vi "MSR Main.vi"() -> ()   [LabVIEW 2019]
uses:
  <vilib>/Platform/TimedLoop/XDataNode/timing_clust.ctl
  <vilib>/Platform/TimedLoop/XDataNode/nitl_modes.ctl
  <vilib>/Platform/TimedLoop/XDataNode/wakeup.ctl
  <vilib>/platform/TimedLoop/XDataNode/XDataNode.xnode
  <vilib>/Platform/TimedLoop/XDataNode/XDNodeRunTimeDep.lvlib
panel:
  in  "Tab Control":enum32{"Plots", "Debug"}(tab)
  out "Flow Plot":cluster{dbl[], dbl[]}(graph)
  out "Temperature Plot":cluster{dbl[], dbl[]}[](graph)
  in  "?":u16(ring)=3 items=["Primary Temperatures", "Secondary Temperatures", "Air Temperatures", "Pri and Sec Temperatures"]
  in  "?":u16(ring) items=["Primary Flow", "Secondary Flow", "Air Flow"]
  out "PriLoops":i32=318
  out "MainLoops":i32=318
  out "SecLoops":i32=318
  out "Time Interval (s)":dbl=0.002
  out "AirLoops":i32=318
  out "Running":bool=TRUE
  out "MHX Heat Transfer (W)":dbl=29227.364495201997 format="%#.0f"
  in  "Period (ms)":i64=2
  out "NDHX Heat Transfer (W)":dbl
  in  "Speed":u16(ring) items=["1x", "10x", "100x", "250x"]
  out "Time Elapsed (s)":dbl=0.6360000000000005
  out "Primary Flow (kg/s)":dbl=0.15588909681163526 format="%.2f"
  out "Primary Cold Temperature (C)":dbl=509.9990851167456 format="%#.1f"
  out "Primary Hot Temperature (C)":dbl=530.011541963479 format="%#.1f"
  out "Primary Ave Temperature (C)":dbl=520.0052977887772 format="%#.1f"
  out "Secondary Flow (kg/s)":dbl=0.18722572734626322 format="%.2f"
  out "Secondary Hot Temperature (C)":dbl=501.012014998414 format="%#.1f"
  out "Secondary Cold Temperature (C)":dbl=490.0008668458488 format="%#.1f"
  out "Secondary Ave Temperature (C)":dbl=495.5064099599597 format="%#.1f"
  out "Air Flow (kg/s)":dbl=0.0013110826649570554 format="%.2f"
  in  "Louver Position (% Open)":dbl=35.0 min=0.0 max=100.0
  in  "Reactor Power (W)":dbl=200000.0 min=0.0 max=250000.0
  out "Air Ave Temperature (C)":dbl=20.007970254732186 format="%#.1f"
  out "Air Outlet Temperature (C)":dbl=20.015996677171586 format="%#.1f"
  in  "Stop":bool
  in  "Air Inlet Temperature (C)":dbl=20.0 min=-89.0 max=57.0
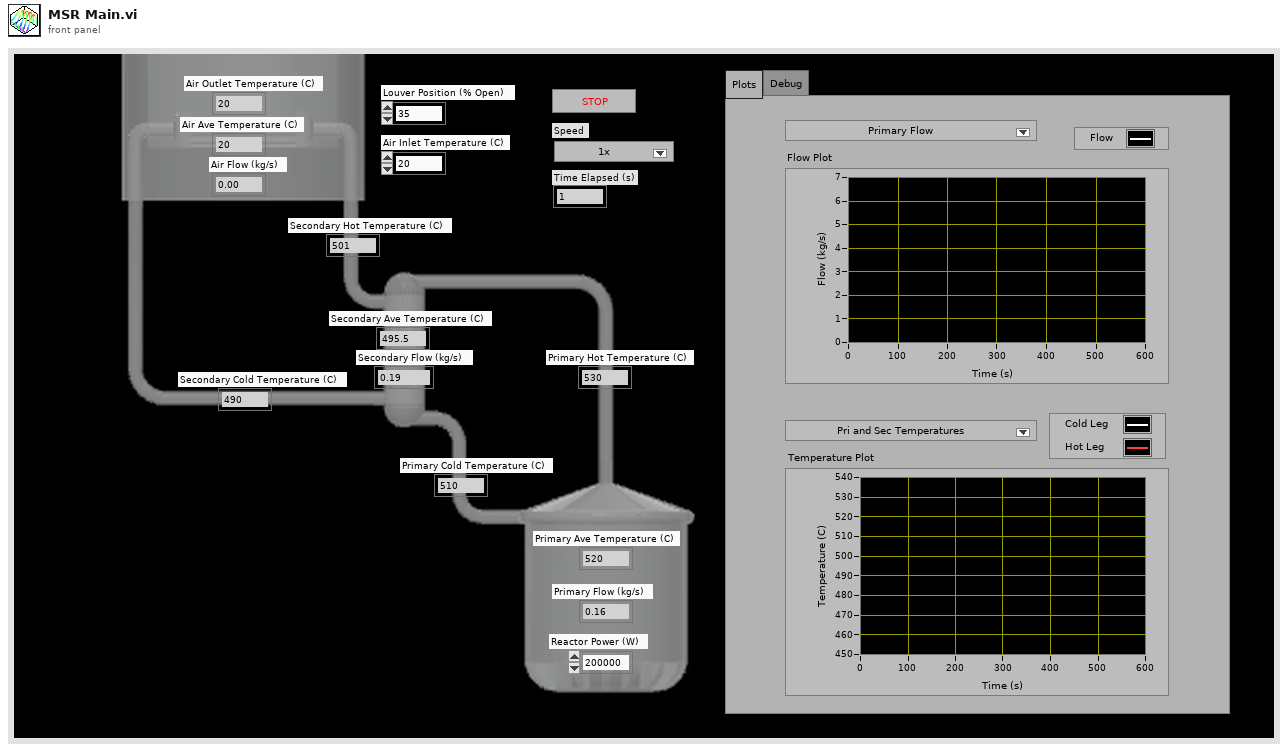
[diagram p1: front panel]
types:
  T1 = cluster{"Air Queue":refnum<queue>, "Air Err":errorcluster, "Pri Queue":refnum<queue>, "Sec Queue":refnum<queue>, "Pri Err":errorcluster, "Sec Err":errorcluster}
  T2 = cluster{"Air Outlet Temperature (K)":dbl, "Air Flow (kg/s)":dbl, "NDHX Wall Temperature (K)":dbl, "Air Visc (Pa-s)":dbl, "Pri Flow (kg/s)":dbl, "Pri Hot Temp (K)":dbl, "Pri Cold Temp (K)":dbl, "Sec Flow (kg/s)":dbl, "Sec Hot Temp (K)":dbl, "Sec Cold Temp (K)":dbl, "MHX Wall Temp (K)":dbl, "FLiNaK Visc (Pa-s)":dbl}
  T3 = cluster{"Pri Flow (kg/s)":dbl, "Pri Hot Temp (K)":dbl, "Pri Cold Temp (K)":dbl}
  T4 = cluster{"Sec Flow (kg/s)":dbl, "Sec Hot Temp (K)":dbl, "Sec Cold Temp (K)":dbl, "MHX Wall Temp (K)":dbl, "FLiNaK Visc (Pa-s)":dbl}
  T5 = typedef "XDNodeRunTimeDep.lvlib/timing_clust.ctl" = cluster{"Expected End [f-1]":u64, "Actual End [f-1]":u64, "Finished Late? [f-1]":bool, "Expected End [i-1]":u64, "Actual End [i-1]":u64, "Finished Late? [i-1]":bool, "Expected Start [i]":u64, "Actual Start [i]":u64, "Expected Start [f]":u64, "Actual Start [f]":u64, "Source Name":string, "Structure Name":string, "Period":i64, "Deadline":i64, "Offset":i64, "Start":i64, "Priority":i32, "Timeout":i32, "Mode":T6, "Wakeup Reason":T7, "Error":errorcluster, "Source Type":string, "Secondary Source Type":string, "Global End Time":u64, "Global Start Time":u64, "Frame Duration":u64, "Iteration Duration":u64, "Assigned CPU":i32, "I/O Scan Engine Mode":u32}
  T6 = typedef "XDNodeRunTimeDep.lvlib/nitl_modes.ctl" = enum32{"No Change", "Process missed periods, maintain original phase", "Discard missed periods, maintain original phase", "Process missed periods, ignore original phase", "Discard missed periods, ignore original phase"}
  T7 = typedef "XDNodeRunTimeDep.lvlib/wakeup.ctl" = enum32{"Normal", "Aborted", "Asynchronous wakeup", "Timing source error", "Timed loop error", "Timeout"}
  T8 = cluster{"Air Outlet Temperature (K)":dbl, "Air Flow (kg/s)":dbl, "NDHX Wall Temperature (K)":dbl, "Air Visc (Pa-s)":dbl}
  T9 = cluster{"Time (s)":dbl, "Air Flow (kg/s)":dbl, "Air Outlet Temp (C)":dbl, "Air Inlet Temp (C)":dbl, "Sec Hot Temp (C)":dbl, "Sec Cold Temp (C)":dbl, "Sec Flow (kg/s)":dbl, "Pri Flow (kg/s)":dbl, "Pri Hot Temp (C)":dbl, "Pri Cold Temp (C)":dbl}
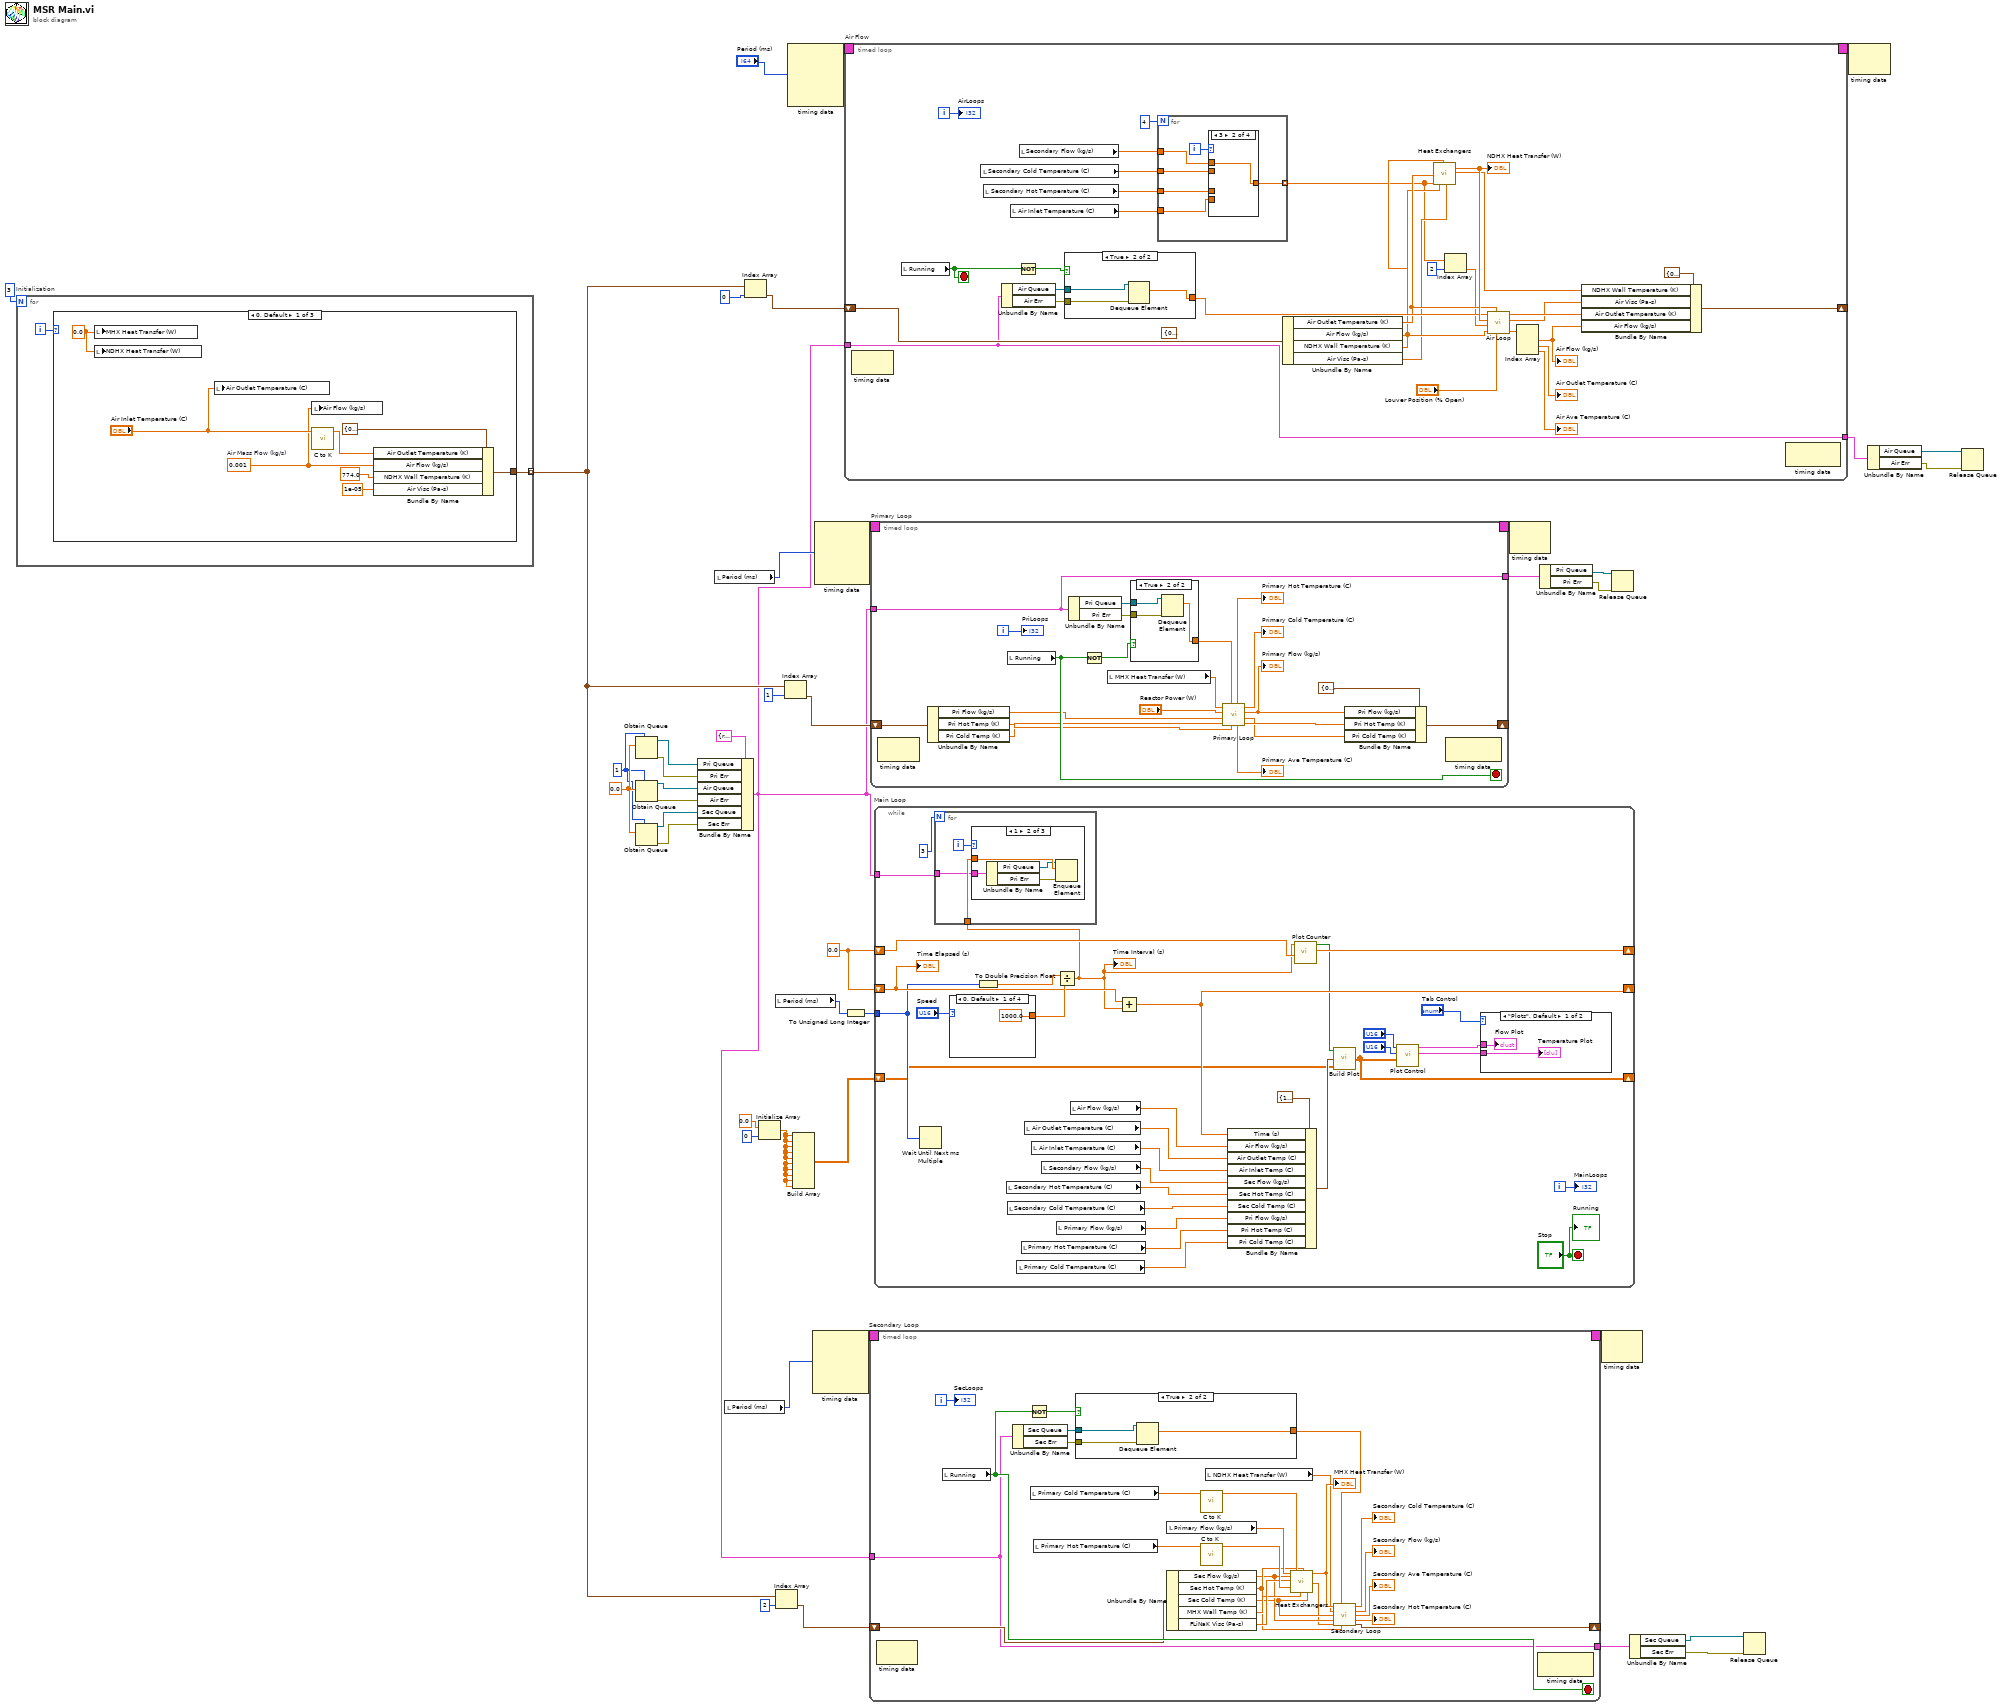
[diagram p0: block diagram]
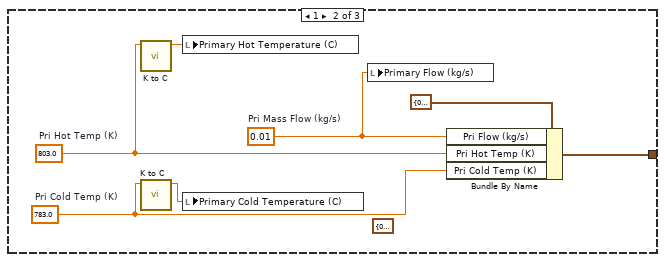
[diagram p2: hidden frame]
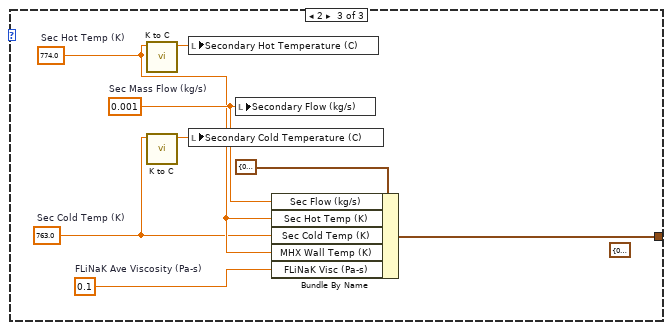
[diagram p3: hidden frame]
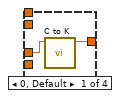
[diagram p4: hidden frame]
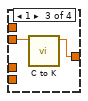
[diagram p5: hidden frame]
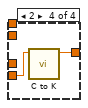
[diagram p6: hidden frame]
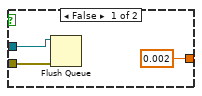
[diagram p7: hidden frame]
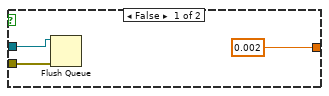
[diagram p8: hidden frame]
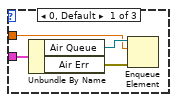
[diagram p9: hidden frame]
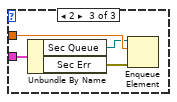
[diagram p10: hidden frame]
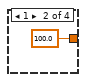
[diagram p12: hidden frame]
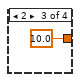
[diagram p13: hidden frame]
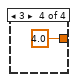
[diagram p14: hidden frame]
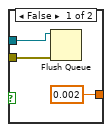
[diagram p15: hidden frame]
diagram:
  w10 = 1 ("max queue size (-1, unlimited)")
  w30 = 0.0
  w35 = 0.0
  n1 = for "Initialization" {
    N: 3 -> [_]
    tunnel: [w45] -> w22 mode=indexing
    i -> [w44]
    n2 = case shown="0, Default" w44 {
      tunnel: [w47 w55 w62] -> w45
      frame 0, Default {
        w46 = 0.0 ("NDHX Heat Transfer (W)")
        w50 = 0.001  # Air Mass Flow (kg/s)
        n3 = local write "MHX Heat Transfer (W)"(w46) -> ()
        n4 = local write "NDHX Heat Transfer (W)"(w46) -> ()
        n5 = local write "Air Outlet Temperature (C)"("Air Inlet Temperature (C)") -> ()
        n6 = local write "Air Flow (kg/s)"(w50) -> ()
        n7 = call "C to K.vi"("Temperature (C)"="Air Inlet Temperature (C)") -> ("Temperature (K)"=w53:dbl)  [unwired: 10 in]
        n8 = Bundle By Name(cluster=T2 {"Air Outlet Temperature (K)"=0.0, "Air Flow (kg/s)"=0.0, "NDHX Wall Temperature (K)"=0.0, "Air Visc (Pa-s)"=0.0, "Pri Flow (kg/s)"=0.0, "Pri Hot Temp (K)"=0.0, "Pri Cold Temp (K)"=0.0, "Sec Flow (kg/s)"=0.0, "Sec Hot Temp (K)"=0.0, "Sec Cold Temp (K)"=0.0, "MHX Wall Temp (K)"=0.0, "FLiNaK Visc (Pa-s)"=0.0} ("input cluster"), "Air Outlet Temperature (K)"=w53, "Air Flow (kg/s)"=w50, "NDHX Wall Temperature (K)"=774.0, "Air Visc (Pa-s)"=1e-05 ("Air Average Viscosity (Pa-s)")) -> (w47:T2)
      }
      frame 1 {
        (unwired) T3 {"Pri Flow (kg/s)"=0.0, "Pri Hot Temp (K)"=0.0, "Pri Cold Temp (K)"=0.0} ("input cluster")
        w58 = 0.01  # Pri Mass Flow (kg/s)
        w56 = 783.0  # Pri Cold Temp (K)
        w57 = 803.0  # Pri Hot Temp (K)
        n9 = call "K to C.vi"("Temperature (K)"=w57) -> ("Temperature (C)"=w60:dbl)  [unwired: 10 in]
        n10 = call "K to C.vi"("Temperature (K)"=w56) -> ("Temperature (C)"=w59:dbl)  [unwired: 10 in]
        n11 = local write "Primary Hot Temperature (C)"(w60) -> ()
        n12 = local write "Primary Cold Temperature (C)"(w59) -> ()
        n13 = local write "Primary Flow (kg/s)"(w58) -> ()
        n14 = Bundle By Name(cluster=T2 {"Air Outlet Temperature (K)"=0.0, "Air Flow (kg/s)"=0.0, "NDHX Wall Temperature (K)"=0.0, "Air Visc (Pa-s)"=0.0, "Pri Flow (kg/s)"=0.0, "Pri Hot Temp (K)"=0.0, "Pri Cold Temp (K)"=0.0, "Sec Flow (kg/s)"=0.0, "Sec Hot Temp (K)"=0.0, "Sec Cold Temp (K)"=0.0, "MHX Wall Temp (K)"=0.0, "FLiNaK Visc (Pa-s)"=0.0} ("input cluster"), "Pri Flow (kg/s)"=w58, "Pri Hot Temp (K)"=w57, "Pri Cold Temp (K)"=w56) -> (w55:T2)
      }
      frame 2 {
        (unwired) T4 {"Sec Flow (kg/s)"=0.0, "Sec Hot Temp (K)"=0.0, "Sec Cold Temp (K)"=0.0, "MHX Wall Temp (K)"=0.0, "FLiNaK Visc (Pa-s)"=0.0} ("input cluster")
        w63 = 0.1  # FLiNaK Ave Viscosity (Pa-s)
        w66 = 0.001  # Sec Mass Flow (kg/s)
        w64 = 763.0  # Sec Cold Temp (K)
        w65 = 774.0  # Sec Hot Temp (K)
        n15 = call "K to C.vi"("Temperature (K)"=w65) -> ("Temperature (C)"=w68:dbl)  [unwired: 10 in]
        n16 = call "K to C.vi"("Temperature (K)"=w64) -> ("Temperature (C)"=w67:dbl)  [unwired: 10 in]
        n17 = local write "Secondary Hot Temperature (C)"(w68) -> ()
        n18 = local write "Secondary Cold Temperature (C)"(w67) -> ()
        n19 = local write "Secondary Flow (kg/s)"(w66) -> ()
        n20 = Bundle By Name(cluster=T2 {"Air Outlet Temperature (K)"=0.0, "Air Flow (kg/s)"=0.0, "NDHX Wall Temperature (K)"=0.0, "Air Visc (Pa-s)"=0.0, "Pri Flow (kg/s)"=0.0, "Pri Hot Temp (K)"=0.0, "Pri Cold Temp (K)"=0.0, "Sec Flow (kg/s)"=0.0, "Sec Hot Temp (K)"=0.0, "Sec Cold Temp (K)"=0.0, "MHX Wall Temp (K)"=0.0, "FLiNaK Visc (Pa-s)"=0.0} ("input cluster"), "Sec Flow (kg/s)"=w66, "Sec Hot Temp (K)"=w65, "Sec Cold Temp (K)"=w64, "MHX Wall Temp (K)"=w65, "FLiNaK Visc (Pa-s)"=w63) -> (w62:T2)
      }
    }
  }
  n21 = Obtain Queue(max queue size (-1, unlimited)=w10, element data type=w35) -> (queue out=w18:refnum<queue>, error out=w17:errorcluster)  [unwired: 3 in, 1 out]
  n22 = Obtain Queue(max queue size (-1, unlimited)=w10, element data type=w35) -> (queue out=w16:refnum<queue>, error out=w15:errorcluster)  [unwired: 3 in, 1 out]
  n23 = Obtain Queue(max queue size (-1, unlimited)=w10, element data type=w35) -> (queue out=w14:refnum<queue>, error out=w13:errorcluster)  [unwired: 3 in, 1 out]
  n24 = Bundle By Name(cluster=T1 {"Air Queue"=refnum, "Air Err"={"status"=FALSE, "code"=0, "source"=""}, "Pri Queue"=refnum, "Sec Queue"=refnum, "Pri Err"={"status"=FALSE, "code"=0, "source"=""}, "Sec Err"={"status"=FALSE, "code"=0, "source"=""}} ("input cluster"), "Pri Queue"=w18, "Pri Err"=w17, "Air Queue"=w16, "Air Err"=w15, "Sec Queue"=w14, "Sec Err"=w13) -> (w11:T1)
  n25 = local read "Period (ms)"() -> (w21:i64)
  n26 = local read "Period (ms)"() -> (w19:i64)
  n27 = Index Array(array=w22, index=0) -> (element=w26:T2)
  n28 = Initialize Array(0.0 ("element"), 0 ("dimension size")) -> (w32:dbl[])
  n29 = local read "Period (ms)"() -> (w20:i64)
  n30 = Index Array(array=w22, index=2) -> (element=w23:T2)
  n31 = Index Array(array=w22, index=1) -> (element=w27:T2)
  n32 = node-c288("Period (ms)") -> (w38:T5)  [unwired: 3 in]
  n33 = Build Array(w32, w32, w32, w32, w32, w32, w32, w32, w32, w32) -> (w31:dbl[][])
  n34 = node-c288(w19) -> (w41:T5)  [unwired: 3 in]
  n35 = node-c288(w21) -> (w43:T5)  [unwired: 3 in]
  n36 = timed-loop "Air Flow" {
    timing: w38 -> [_]
    timing-out: [_] -> w37
    shift-right: [w80] -> _
    shift-left: w26 -> [w93]
    tunnel: w11 -> [w77]
    tunnel: [w77] -> w7
    i -> [w99]
    stop <- w96 stop-if-true
    (unwired) T8 {"Air Outlet Temperature (K)"=0.0, "Air Flow (kg/s)"=0.0, "NDHX Wall Temperature (K)"=0.0, "Air Visc (Pa-s)"=0.0} ("input cluster")
    n37 = node-c288() -> ()  [unwired: 1 in, 1 out]
    n38 = local read "Running"() -> (w96:bool)
    n39 = local read "Secondary Cold Temperature (C)"() -> (w87:dbl)
    n40 = local read "Secondary Hot Temperature (C)"() -> (w88:dbl)
    n41 = Unbundle By Name(w77) -> ("Air Queue"=w79:refnum<queue>, "Air Err"=w78:errorcluster)
    n42 = local read "Air Inlet Temperature (C)"() -> (w86:dbl)
    n43 = Not(x=w96) -> (.not. x?=w98:bool)
    n44 = local read "Secondary Flow (kg/s)"() -> (w69:dbl)
    n45 = case shown="True" w98 {
      tunnel: w79 -> [w115 w117]
      tunnel: w78 -> [w114 w116]
      tunnel: [0.002 w118] -> w94
      frame False {
        n46 = Flush Queue(queue=w115, error in (no error)=w114) -> ()  [unwired: 3 out]
      }
      frame True {
        n47 = Dequeue Element(queue=w117, error in (no error)=w116) -> (element=w118:dbl)  [unwired: 1 in, 3 out]
      }
    }
    n48 = for {
      N: 4 -> [_]
      tunnel: w88 -> [w104]
      tunnel: w87 -> [w102]
      tunnel: w86 -> [w101]
      tunnel: [w103] -> w82 mode=indexing
      tunnel: w69 -> [w100]
      i -> [w105]
      n49 = case shown="3" w105 {
        tunnel: w104 -> [w107 _ _ _]
        tunnel: [w106 w108 w109 w111] -> w103
        tunnel: w102 -> [_ _ w110 _]
        tunnel: w101 -> [_ _ _ w112]
        tunnel: w100 -> [_ w108 _ _]
        frame 0, Default {
          n50 = call "C to K.vi"("Temperature (C)"=w107) -> ("Temperature (K)"=w106:dbl)  [unwired: 10 in]
        }
        frame 3 {
        }
        frame 1 {
          n51 = call "C to K.vi"("Temperature (C)"=w110) -> ("Temperature (K)"=w109:dbl)  [unwired: 10 in]
        }
        frame 2 {
          n52 = call "C to K.vi"("Temperature (C)"=w112) -> ("Temperature (K)"=w111:dbl)  [unwired: 10 in]
        }
      }
    }
    n53 = Unbundle By Name(w93) -> ("Air Outlet Temperature (K)"=w92:dbl, "Air Flow (kg/s)"=w91:dbl, "NDHX Wall Temperature (K)"=w90:dbl, "Air Visc (Pa-s)"=w89:dbl)
    n54 = call "Heat Exchangers.vi"("Air Hot Temperature (K), N"=w92, "Local Array In, N"=w82, "NDHX Tube Wall Temp (K), N"=w90, "Air Flow (kg/s), N"=w91, "Air Average Viscosity (Pa-s), N"=w89) -> ("NDHX Heating Transfer (W)"=w95:dbl, "NDHX Tube Wall Temperature (K)"=w76:dbl)  [unwired: 11 in, 2 out]
    "NDHX Heat Transfer (W)" <- w95
    n55 = Index Array(array=w82, index=2) -> (element=w83:dbl)
    n56 = call "Air Loop.vi"("Louver Position (% Open)"="Louver Position (% Open)", "Air Hot Temperature (K)"=w92, "Air Mass Flow (kg/s) in"=w91, "Air Inlet Temperature (K)"=w83, "NDHX Heat Transfer (W)"=w95, "Time Interval (s)"=w94) -> ("Indications"=w75:dbl[], "Air Average Viscosity (Pa-s)"=w71:dbl, "Air Outlet Temperature (K)"=w72:dbl)  [unwired: 2 in, 1 out]
    n57 = Index Array(array=w75) -> (element #1=w70:dbl, element #2=→"Air Outlet Temperature (C)":dbl, element #3=→"Air Ave Temperature (C)":dbl)  [unwired: 3 in]
    "Air Flow (kg/s)" <- w70
    n58 = Bundle By Name(cluster=T2 {"Air Outlet Temperature (K)"=0.0, "Air Flow (kg/s)"=0.0, "NDHX Wall Temperature (K)"=0.0, "Air Visc (Pa-s)"=0.0, "Pri Flow (kg/s)"=0.0, "Pri Hot Temp (K)"=0.0, "Pri Cold Temp (K)"=0.0, "Sec Flow (kg/s)"=0.0, "Sec Hot Temp (K)"=0.0, "Sec Cold Temp (K)"=0.0, "MHX Wall Temp (K)"=0.0, "FLiNaK Visc (Pa-s)"=0.0} ("input cluster"), "NDHX Wall Temperature (K)"=w76, "Air Visc (Pa-s)"=w71, "Air Outlet Temperature (K)"=w72, "Air Flow (kg/s)"=w70) -> (w80:T2)
    n59 = node-c288() -> ()  [unwired: 1 in, 1 out]
    "AirLoops" <- w99
  }
  n60 = To Unsigned Long Integer(number=w20) -> (unsigned 32bit integer=w39:u32)
  n61 = timed-loop "Secondary Loop" {
    timing: w41 -> [_]
    timing-out: [_] -> w40
    shift-right: [w125] -> _
    shift-left: w23 -> [w134]
    tunnel: w11 -> [w122]
    tunnel: [w122] -> w3
    i -> [w146]
    stop <- w144 stop-if-true
    n62 = node-c288() -> ()  [unwired: 1 in, 1 out]
    n63 = local read "Running"() -> (w144:bool)
    n64 = Unbundle By Name(w122) -> ("Sec Queue"=w124:refnum<queue>, "Sec Err"=w123:errorcluster)
    n65 = Not(x=w144) -> (.not. x?=w143:bool)
    n66 = local read "Primary Cold Temperature (C)"() -> (w140:dbl)
    n67 = local read "Primary Hot Temperature (C)"() -> (w141:dbl)
    n68 = case shown="True" w143 {
      tunnel: w124 -> [w149 w152]
      tunnel: w123 -> [w148 w151]
      tunnel: [0.002 w150] -> w136
      frame False {
        n69 = Flush Queue(queue=w149, error in (no error)=w148) -> ()  [unwired: 3 out]
      }
      frame True {
        n70 = Dequeue Element(queue=w152, error in (no error)=w151) -> (element=w150:dbl)  [unwired: 1 in, 3 out]
      }
    }
    n71 = local read "Primary Flow (kg/s)"() -> (w142:dbl)
    n72 = Unbundle By Name(w134) -> ("Sec Flow (kg/s)"=w130:dbl, "Sec Hot Temp (K)"=w131:dbl, "Sec Cold Temp (K)"=w129:dbl, "MHX Wall Temp (K)"=w132:dbl, "FLiNaK Visc (Pa-s)"=w133:dbl)
    n73 = call "C to K.vi"("Temperature (C)"=w140) -> ("Temperature (K)"=w139:dbl)  [unwired: 10 in]
    n74 = call "C to K.vi"("Temperature (C)"=w141) -> ("Temperature (K)"=w138:dbl)  [unwired: 10 in]
    n75 = local read "NDHX Heat Transfer (W)"() -> (w121:dbl)
    n76 = call "Heat Exchangers.vi"("Primary Flow (kg/s), M"=w142, "Secondary Flow (kg/s)"=w130, "FLiNaK Ave Viscosity (Pa-s), M"=w133, "Pri Hot Temperature (K), M"=w138, "Pri Cold Temperature (K), M"=w139, "MHX Tube Wall Temp (K), M"=w132, "Sec Hot Temperature (K)"=w131, "Sec Cold Temperature (K)"=w129) -> ("MHX Heat Transfer (W)"=w137:dbl, "MHX Tube Wall Temperature (K)"=w128:dbl)  [unwired: 8 in, 2 out]
    "MHX Heat Transfer (W)" <- w137
    n77 = call "Secondary Loop.vi"("MHX Heat Transfer (W)"=w137, "Time Interval (s)"=w136, "NDHX Heat Transfer (W)"=w121, "Sec Cold Temp (K)"=w129, "Sec Mass Flow (kg/s) in"=w130, "MHX Wall Temp (K)"=w128, "Sec Hot Temp (K) in"=w131) -> ("Sec Cold Temperature (C)"=→"Secondary Cold Temperature (C)":dbl, "Sec Mass Flow (kg/s) out"=→"Secondary Flow (kg/s)":dbl, "Secondary Average Temperature (C)"=→"Secondary Ave Temperature (C)":dbl, "Sec Hot Temperature (C)"=→"Secondary Hot Temperature (C)":dbl, "output cluster"=w125:T2)  [unwired: 4 in]
    n78 = node-c288() -> ()  [unwired: 1 in, 1 out]
    "SecLoops" <- w146
  }
  n79 = timed-loop "Primary Loop" {
    timing: w43 -> [_]
    timing-out: [_] -> w42
    shift-right: [w158] -> _
    shift-left: w27 -> [w163]
    tunnel: w11 -> [w155]
    tunnel: [w155] -> w6
    i -> [w175]
    stop <- w170 stop-if-true
    n80 = node-c288() -> ()  [unwired: 1 in, 1 out]
    n81 = Unbundle By Name(w163) -> ("Pri Flow (kg/s)"=w162:dbl, "Pri Hot Temp (K)"=w161:dbl, "Pri Cold Temp (K)"=w160:dbl)
    n82 = local read "Running"() -> (w170:bool)
    n83 = Unbundle By Name(w155) -> ("Pri Queue"=w157:refnum<queue>, "Pri Err"=w156:errorcluster)
    n84 = Not(x=w170) -> (.not. x?=w169:bool)
    n85 = local read "MHX Heat Transfer (W)"() -> (w168:dbl)
    n86 = case shown="True" w169 {
      tunnel: w157 -> [w178 w180]
      tunnel: w156 -> [w177 w179]
      tunnel: [0.002 w181] -> w167
      frame False {
        n87 = Flush Queue(queue=w178, error in (no error)=w177) -> ()  [unwired: 3 out]
      }
      frame True {
        n88 = Dequeue Element(queue=w180, error in (no error)=w179) -> (element=w181:dbl)  [unwired: 1 in, 3 out]
      }
    }
    n89 = call "Primary Loop.vi"("Pri Hot Temp (K)"=w161, "Time Interval (s)"=w167, "Pri Cold Temp (K)"=w160, "Pri Mass Flow (kg/s) in"=w162, "Reactor Power (W)"="Reactor Power (W)", "MHX Heat Transfer (W)"=w168) -> ("Pri Hot Temperature (K)"=w165:dbl, "Pri Cold Temperature (K)"=w164:dbl, "Pri Mass Flow (kg/s) out"=w166:dbl, "Temperature (C) 2"=→"Primary Cold Temperature (C)":dbl, "Primary Average Temperature (C)"=→"Primary Ave Temperature (C)":dbl, "Temperature (C)"=→"Primary Hot Temperature (C)":dbl)
    "Primary Flow (kg/s)" <- w166
    n90 = Bundle By Name(cluster=T2 {"Air Outlet Temperature (K)"=0.0, "Air Flow (kg/s)"=0.0, "NDHX Wall Temperature (K)"=0.0, "Air Visc (Pa-s)"=0.0, "Pri Flow (kg/s)"=0.0, "Pri Hot Temp (K)"=0.0, "Pri Cold Temp (K)"=0.0, "Sec Flow (kg/s)"=0.0, "Sec Hot Temp (K)"=0.0, "Sec Cold Temp (K)"=0.0, "MHX Wall Temp (K)"=0.0, "FLiNaK Visc (Pa-s)"=0.0} ("input cluster"), "Pri Flow (kg/s)"=w166, "Pri Hot Temp (K)"=w165, "Pri Cold Temp (K)"=w164) -> (w158:T2)
    n91 = node-c288() -> ()  [unwired: 1 in, 1 out]
    "PriLoops" <- w175
  }
  n92 = while "Main Loop" {
    shift-right: [w200] -> _
    shift-left: w30 -> [w212]
    shift-right: [w208] -> _
    shift-left: w30 -> [w203]
    tunnel: w39 -> [w207]
    shift-right: [w186] -> _
    shift-left: w31 -> [w187]
    tunnel: w11 -> [w185]
    i -> [w209]
    stop <- "Stop" stop-if-true
    n93 = Wait Until Next ms Multiple(millisecond multiple=w207) -> ()  [unwired: 1 out]
    n94 = case shown="0, Default" "Speed" {
      tunnel: [1000.0 100.0 ("y") 10.0 ("y") 4.0 ("y")] -> w213
      frame 0, Default {
      }
      frame 1 {
      }
      frame 2 {
      }
      frame 3 {
      }
    }
    n95 = To Double Precision Float(number=w207) -> (double precision float=w215:dbl)
    n96 = local read "Secondary Hot Temperature (C)"() -> (w195:dbl)
    n97 = local read "Secondary Cold Temperature (C)"() -> (w194:dbl)
    n98 = local read "Primary Cold Temperature (C)"() -> (w191:dbl)
    n99 = local read "Primary Hot Temperature (C)"() -> (w192:dbl)
    n100 = local read "Air Outlet Temperature (C)"() -> (w198:dbl)
    n101 = local read "Air Inlet Temperature (C)"() -> (w197:dbl)
    n102 = local read "Secondary Flow (kg/s)"() -> (w196:dbl)
    n103 = Divide(x=w215, y=w213) -> (x/y=w202:dbl)
    "Time Interval (s)" <- w202
    n104 = for {
      N: 3 -> [_]
      tunnel: w202 -> [w218]
      tunnel: w185 -> [w217]
      i -> [w216]
      n105 = case shown="1" w216 {
        tunnel: w218 -> [w219 w226 w230]
        tunnel: w217 -> [w220 w225 w229]
        frame 0, Default {
          n106 = Unbundle By Name(w220) -> ("Air Queue"=w222:refnum<queue>, "Air Err"=w221:errorcluster)
          n107 = Enqueue Element(queue=w222, element=w219, error in (no error)=w221) -> ()  [unwired: 1 in, 3 out]
        }
        frame 1 {
          n108 = Unbundle By Name(w225) -> ("Pri Queue"=w224:refnum<queue>, "Pri Err"=w223:errorcluster)
          n109 = Enqueue Element(queue=w224, element=w226, error in (no error)=w223) -> ()  [unwired: 1 in, 3 out]
        }
        frame 2 {
          n110 = Unbundle By Name(w229) -> ("Sec Queue"=w228:refnum<queue>, "Sec Err"=w227:errorcluster)
          n111 = Enqueue Element(queue=w228, element=w230, error in (no error)=w227) -> ()  [unwired: 1 in, 3 out]
        }
      }
    }
    n112 = local read "Primary Flow (kg/s)"() -> (w193:dbl)
    n113 = local read "Air Flow (kg/s)"() -> (w199:dbl)
    n114 = Add(x=w212, y=w202) -> (x+y=w200:dbl)
    n115 = Bundle By Name(cluster=T9 {"Time (s)"=1000.0, "Air Flow (kg/s)"=1000.0, "Air Outlet Temp (C)"=1000.0, "Air Inlet Temp (C)"=1000.0, "Sec Hot Temp (C)"=1000.0, "Sec Cold Temp (C)"=1000.0, "Sec Flow (kg/s)"=1000.0, "Pri Flow (kg/s)"=1000.0, "Pri Hot Temp (C)"=1000.0, "Pri Cold Temp (C)"=1000.0} ("input cluster"), "Time (s)"=w200, "Air Flow (kg/s)"=w199, "Air Outlet Temp (C)"=w198, "Air Inlet Temp (C)"=w197, "Sec Flow (kg/s)"=w196, "Sec Hot Temp (C)"=w195, "Sec Cold Temp (C)"=w194, "Pri Flow (kg/s)"=w193, "Pri Hot Temp (C)"=w192, "Pri Cold Temp (C)"=w191) -> (w188:T9)
    n116 = call "Plot Counter.vi"("y in"=w203, "Numeric"=w202) -> ("y out"=w208:dbl, "Boolean out"=w189:bool)  [unwired: 8 in]
    n117 = call "Build Plot.vi"("Array in"=w187, "Data cluster"=w188, "Boolean in"=w189) -> ("Array out"=w186:dbl[][])
    n118 = call "Plot Control.vi"("Data"=w186, "Temperature Selection"="?", "Flow Selection"="?") -> ("Temperature Plot"=w204:cluster{"Array out":dbl[], "Array out":dbl[]}[], "Flow Plot"=w205:cluster{"Array out":dbl[], "Array out":dbl[]})  [unwired: 7 in]
    n119 = case shown="\"Plots\", Default" "Tab Control" {
      tunnel: w205 -> [w232 _]
      tunnel: w204 -> [w231 _]
      frame "Plots", Default {
        "Flow Plot" <- w232
        "Temperature Plot" <- w231
      }
      frame "Debug" {
      }
    }
    "Time Elapsed (s)" <- w212
    "MainLoops" <- w209
    "Running" <- "Stop"
  }
  n120 = node-c288(w42) -> ()  [unwired: 1 out]
  n121 = Unbundle By Name(w6) -> ("Pri Queue"=w5:refnum<queue>, "Pri Err"=w4:errorcluster)
  n122 = node-c288(w40) -> ()  [unwired: 1 out]
  n123 = Release Queue(queue=w5, error in (no error)=w4) -> ()  [unwired: 1 in, 3 out]
  n124 = Unbundle By Name(w3) -> ("Sec Queue"=w2:refnum<queue>, "Sec Err"=w1:errorcluster)
  n125 = Release Queue(queue=w2, error in (no error)=w1) -> ()  [unwired: 1 in, 3 out]
  n126 = node-c288(w37) -> ()  [unwired: 1 out]
  n127 = Unbundle By Name(w7) -> ("Air Queue"=w9:refnum<queue>, "Air Err"=w8:errorcluster)
  n128 = Release Queue(queue=w9, error in (no error)=w8) -> ()  [unwired: 1 in, 3 out]
